vi "CBC加密.vi"(8 "error in (no error)":errorcluster caption="错误输入（无错误）", 9 "IV":string="78352310323ABCDE", 10 "钥匙":string="78352310323ABCDE", 11 "明文":string="abcdefghijklmnopabcdefghijklmno") -> (0 "error out":errorcluster caption="错误输出", 3 "密文":string)   [LabVIEW 2016, in "数据传输系统-02.lvlib"]
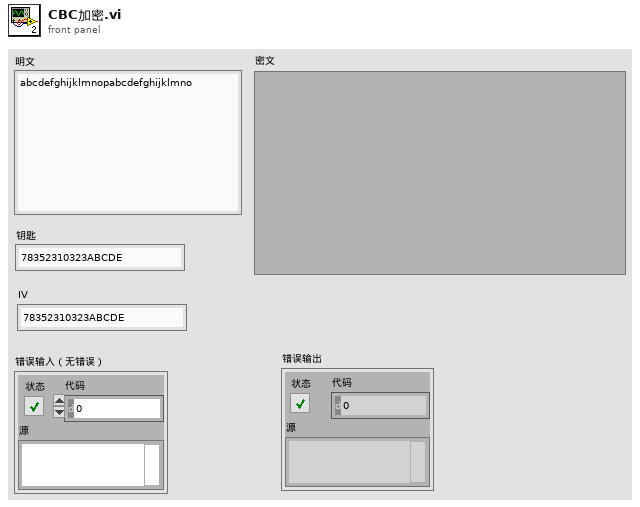
[diagram p1: front panel]
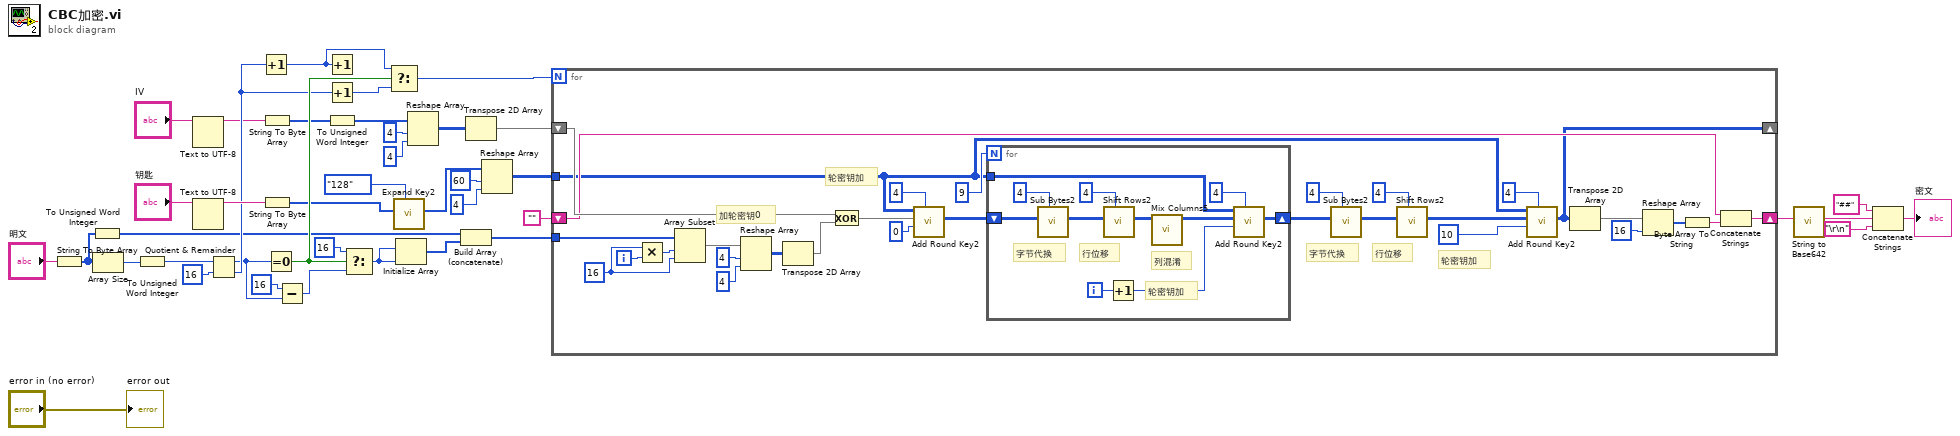
[diagram p0: block diagram]
diagram:
  n1 = String To Byte Array(string="明文") -> (unsigned byte array=w27:u8[])
  n2 = To Unsigned Word Integer(number=w27) -> (unsigned 16bit integer=w26:u16[])
  n3 = Array Size(array=w27) -> (size(s)=w25:i32)
  n4 = To Unsigned Word Integer(number=w25) -> (unsigned 16bit integer=w23:u16)
  n5 = Text to UTF-8(11:"IV") -> (3:w8:string)  [unwired: 2 in, 1 out]
  n6 = Text to UTF-8(11:"钥匙") -> (3:w40:string)  [unwired: 2 in, 1 out]
  n7 = Quotient & Remainder(x=w23, y=u16 16) -> (x-y*floor(x/y)=w21:u16, floor(x/y)=w29:u16)
  n8 = Increment(x=w29) -> (x+1=w1:u16)
  n9 = String To Byte Array(string=w8) -> (unsigned byte array=w7:u8[])
  n10 = String To Byte Array(string=w40) -> (unsigned byte array=w11:u8[])
  n11 = Equal To 0?(x=w21) -> (x = 0?=w32:bool)
  n12 = Subtract(x=u16 16 ("元素"), y=w21) -> (x-y=w20:u16)
  n13 = Increment(x=w1) -> ()  [unwired: 1 out]
  n14 = Increment(x=w29) -> (x+1=w30:u16)
  n15 = To Unsigned Word Integer(number=w7) -> (unsigned 16bit integer=w28:u16[])
  n16 = Select(t=u16 16 ("元素"), s=w32, f=w20) -> (s? t:f=w33:u16)
  n17 = Select(t=w1, s=w32, f=w30) -> (s? t:f=w18:u16)
  n18 = call "Expand Key2.vi"("Mode (auto)"=enum16{"128", "192", "256", "auto"}."128", "Key"=w11) -> ("Expanded Key"=w15:u32[])  [unwired: 8 in, 1 out]
  n19 = Initialize Array(w33, w33) -> (w19:u16[])
  n20 = Reshape Array(w28, 4 ("dimension size"), 4 ("dimension size")) -> (w37:u16[][])
  n21 = Build Array (concatenate)(w26, w19) -> (w36:u16[])
  n22 = Transpose 2D Array(2D array=w37) -> (transposed array=w17:u16[][])
  n23 = Reshape Array(w15, 60 ("dimension size"), 4 ("dimension size")) -> (w10:u32[][])
  n24 = for {
    N: w18 -> [_]
    tunnel: w36 -> [w49]
    shift-right: [w50] -> w41
    shift-left: "" -> [w51]
    shift-right: [w43] -> _
    shift-left: w17 -> [w55]
    tunnel: w10 -> [w42]
    i -> [w48]
    w47 = 16 ("元素")
    # "轮密钥加"
    # "轮密钥加"
    # "行位移"
    # "字节代换"
    # "加轮密钥0"
    n25 = Multiply(x=w47, y=w48) -> (x*y=w46:i32)
    n26 = Array Subset(array=w49, index=w46, length=w47) -> (w45:u16[])
    n27 = Reshape Array(w45, 4 ("dimension size"), 4 ("dimension size")) -> (w69:u16[][])
    n28 = Transpose 2D Array(2D array=w69) -> (transposed array=w54:u16[][])
    n29 = Exclusive Or(1:w54, 2:w55) -> (0:w53:u16[][])
    n30 = call "Add Round Key2.vi"("Nb"=4, "rnd (0)"=0, "State.In"=w53, "ExpandedKey(w)"=w42) -> ("State.Out"=w66:u16[][])  [unwired: 6 in, 1 out]
    n31 = for {
      N: 9 -> [_]
      tunnel: w42 -> [w77]
      shift-right: [w74] -> w61
      shift-left: w66 -> [w78]
      i -> [w73]
      # "轮密钥加"
      # "列混淆"
      # "行位移"
      # "字节代换"
      n32 = call "Sub Bytes2.vi"("Nb"=4, "State In"=w78) -> ("State Out"=w81:u16[][])  [unwired: 8 in, 1 out]
      n33 = call "Shift Rows2.vi"("Nb"=4, "State In"=w81) -> ("State Out"=w79:u16[][])  [unwired: 8 in, 1 out]
      n34 = Increment(x=w73) -> (x+1=w72:i32)
      n35 = call "Mix Columns5.vi"("State In"=w79) -> ("数组"=w76:u16[][])  [unwired: 10 in]
      n36 = call "Add Round Key2.vi"("Nb"=4, "rnd (0)"=w72, "State.In"=w76, "ExpandedKey(w)"=w77) -> ("State.Out"=w74:u16[][])  [unwired: 6 in, 1 out]
    }
    n37 = call "Sub Bytes2.vi"("Nb"=4, "State In"=w61) -> ("State Out"=w63:u16[][])  [unwired: 8 in, 1 out]
    n38 = call "Shift Rows2.vi"("Nb"=4, "State In"=w63) -> ("State Out"=w58:u16[][])  [unwired: 8 in, 1 out]
    n39 = call "Add Round Key2.vi"("Nb"=4, "rnd (0)"=10, "State.In"=w58, "ExpandedKey(w)"=w42) -> ("State.Out"=w43:u16[][])  [unwired: 6 in, 1 out]
    n40 = Transpose 2D Array(2D array=w43) -> (transposed array=w44:u16[][])
    n41 = Reshape Array(w44, 16 ("维数大小")) -> (w56:u16[])
    n42 = Byte Array To String(unsigned byte array=w56) -> (string=w52:string)
    n43 = Concatenate Strings(w51, w52) -> (w50:string)
  }
  n44 = call "String to Base642.vi"("Plain String"=w41) -> ("Base64 String"=w2:string)  [unwired: 9 in, 1 out]
  n45 = Concatenate Strings("##", w2, "\r\n") -> (→"密文":string)
  "error out" <- "error in (no error)"
